vi "Import OBJ.vi"(8 "error in (no error)":errorcluster, 11 "Object":path) -> (0 "error out":errorcluster, 3 "Object":T8 {"Triangles"."Vertex 3"."UV"."v" min=0 max=1 step=0.1; "Triangles"."Vertex 3"."UV"."u" min=0 max=1 step=0.1; "Triangles"."Vertex 2"."UV"."v" min=0 max=1 step=0.1; "Triangles"."Vertex 2"."UV"."u" min=0 max=1 step=0.1; "Triangles"."Vertex 1"."UV"."v" min=0 max=1 step=0.1; "Triangles"."Vertex 1"."UV"."u" min=0 max=1 step=0.1})   [LabVIEW 2020, in "3D (FPGA).lvlib"]
uses:
  3D (FPGA).lvlib
  Vector 3D.ctl
  Object.ctl
  Transform.ctl
  Raster/UV.ctl
  Raster/Raster (FPGA).lvlib
  Vertex.ctl
  Triangle.ctl
  Raster/Rectangle Dimensions.ctl
  Raster/Texture.ctl
  Material.ctl
panel:
  out "Tris":T1[](array[typedef]) {"Vertex 3"."UV"."v" min=0 max=1 step=0.1; "Vertex 3"."UV"."u" min=0 max=1 step=0.1; "Vertex 2"."UV"."v" min=0 max=1 step=0.1; "Vertex 2"."UV"."u" min=0 max=1 step=0.1; "Vertex 1"."UV"."v" min=0 max=1 step=0.1; "Vertex 1"."UV"."u" min=0 max=1 step=0.1}
  out "text":string[](array[string])
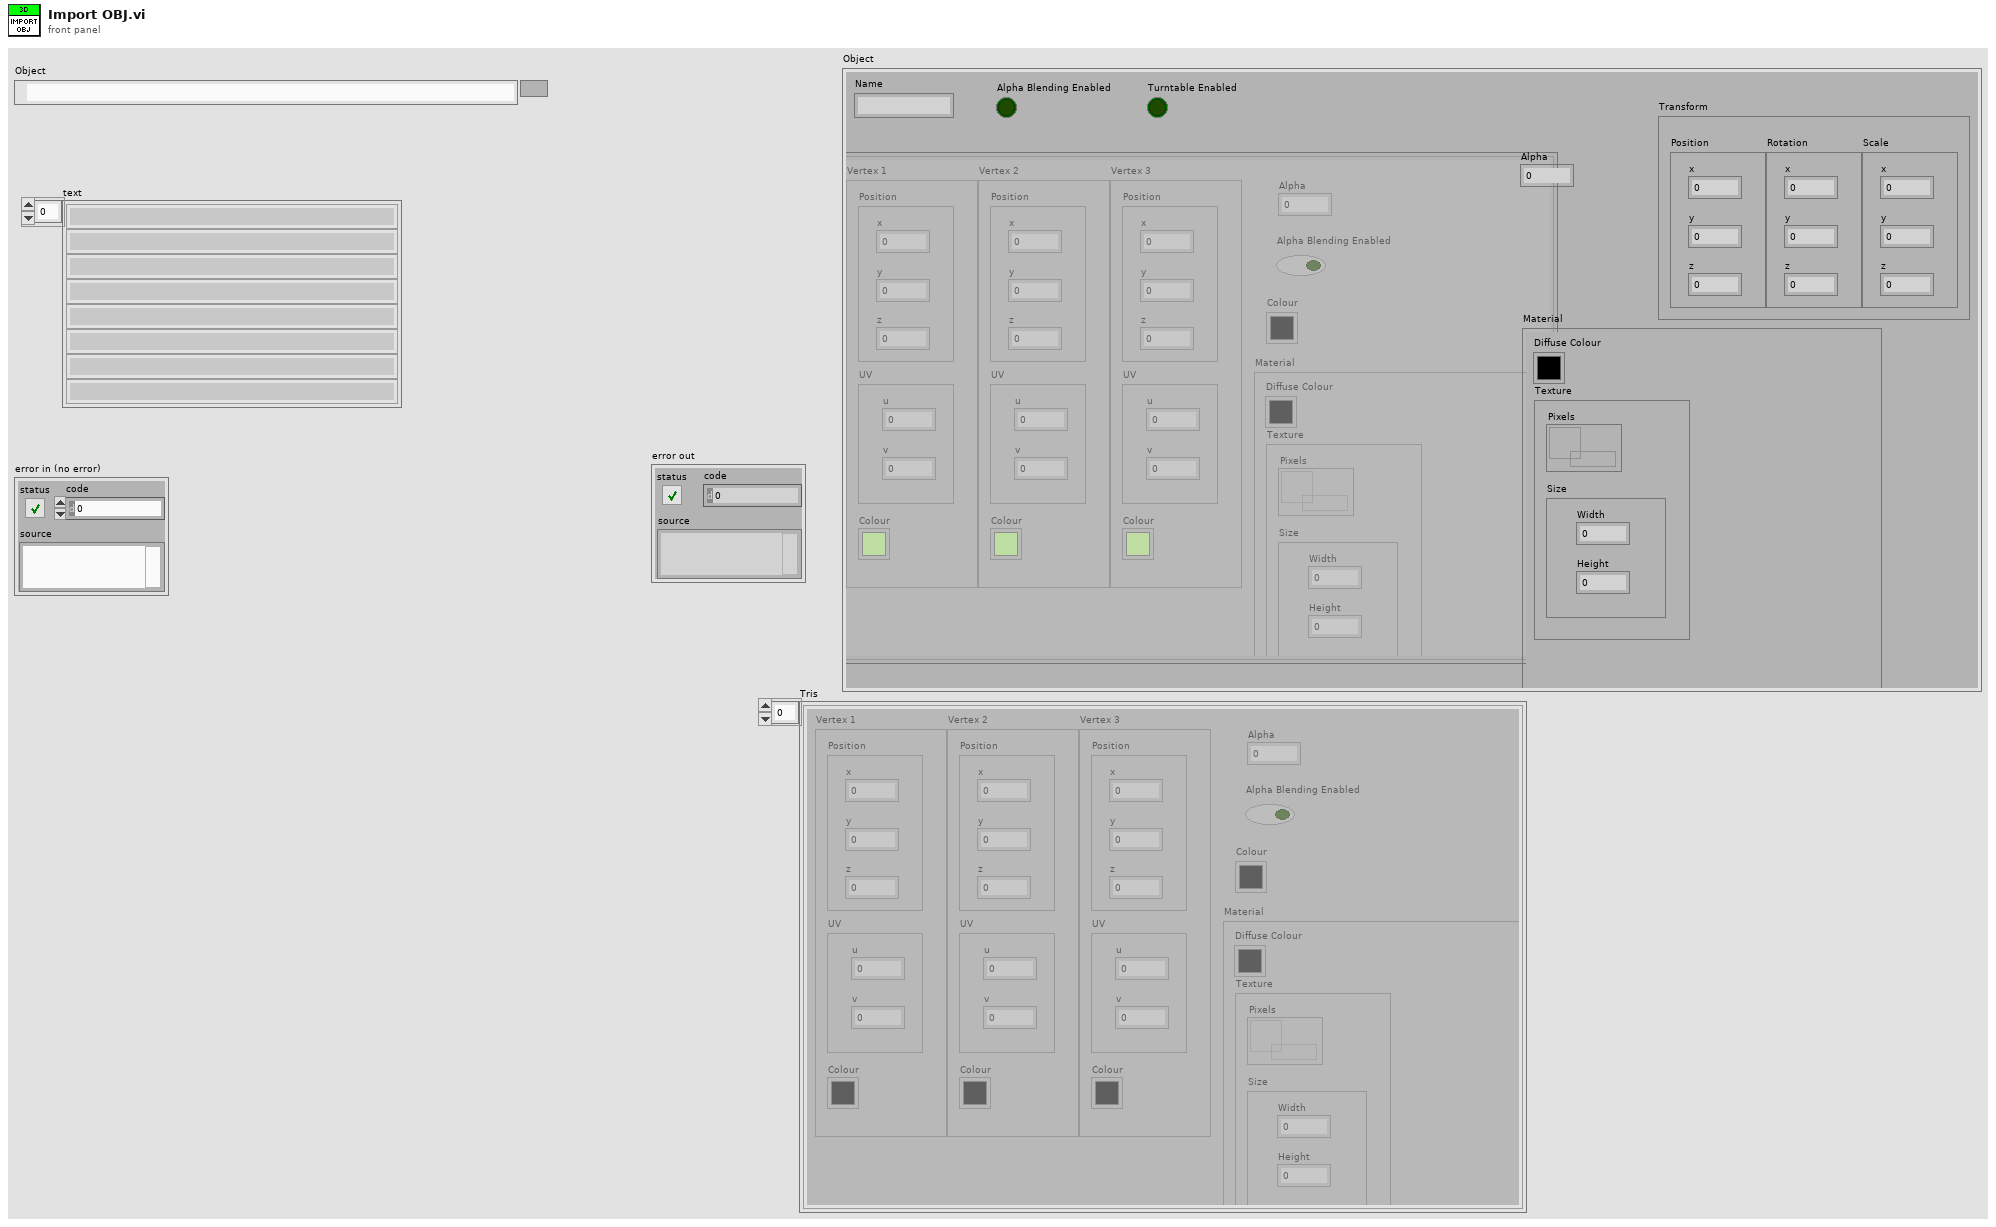
[diagram p1: front panel]
types:
  T1 = typedef "3D (FPGA).lvlib/Triangle.ctl" = cluster{"Vertex 1":T2, "Vertex 2":T2, "Vertex 3":T2, "Alpha":dbl, "Alpha Blending Enabled":bool, "Colour":u32, "Material":T5}
  T2 = typedef "3D (FPGA).lvlib/Vertex.ctl" = cluster{"Position":T3, "UV":T4, "Colour":u32}
  T3 = typedef "3D (FPGA).lvlib/Vector 3D.ctl" = cluster{"x":sgl, "y":sgl, "z":sgl}
  T4 = typedef "Raster (FPGA).lvlib/UV.ctl" = cluster{"u":sgl, "v":sgl}
  T5 = typedef "3D (FPGA).lvlib/Material.ctl" = cluster{"Diffuse Colour":u32, "Texture":T6}
  T6 = typedef "Raster (FPGA).lvlib/Texture.ctl" = cluster{"Pixels":refnum<data-value>, "Size":T7}
  T7 = typedef "Raster (FPGA).lvlib/Rectangle Dimensions.ctl" = cluster{"Width":u32, "Height":u32}
  T8 = typedef "3D (FPGA).lvlib/Object.ctl" = cluster{"Triangles":T1[], "Transform":T9, "Name":string, "Alpha Blending Enabled":bool, "Alpha":dbl, "Turntable Enabled":bool, "Material":T5}
  T9 = typedef "3D (FPGA).lvlib/Transform.ctl" = cluster{"Position":T3, "Rotation":T3, "Scale":T3}
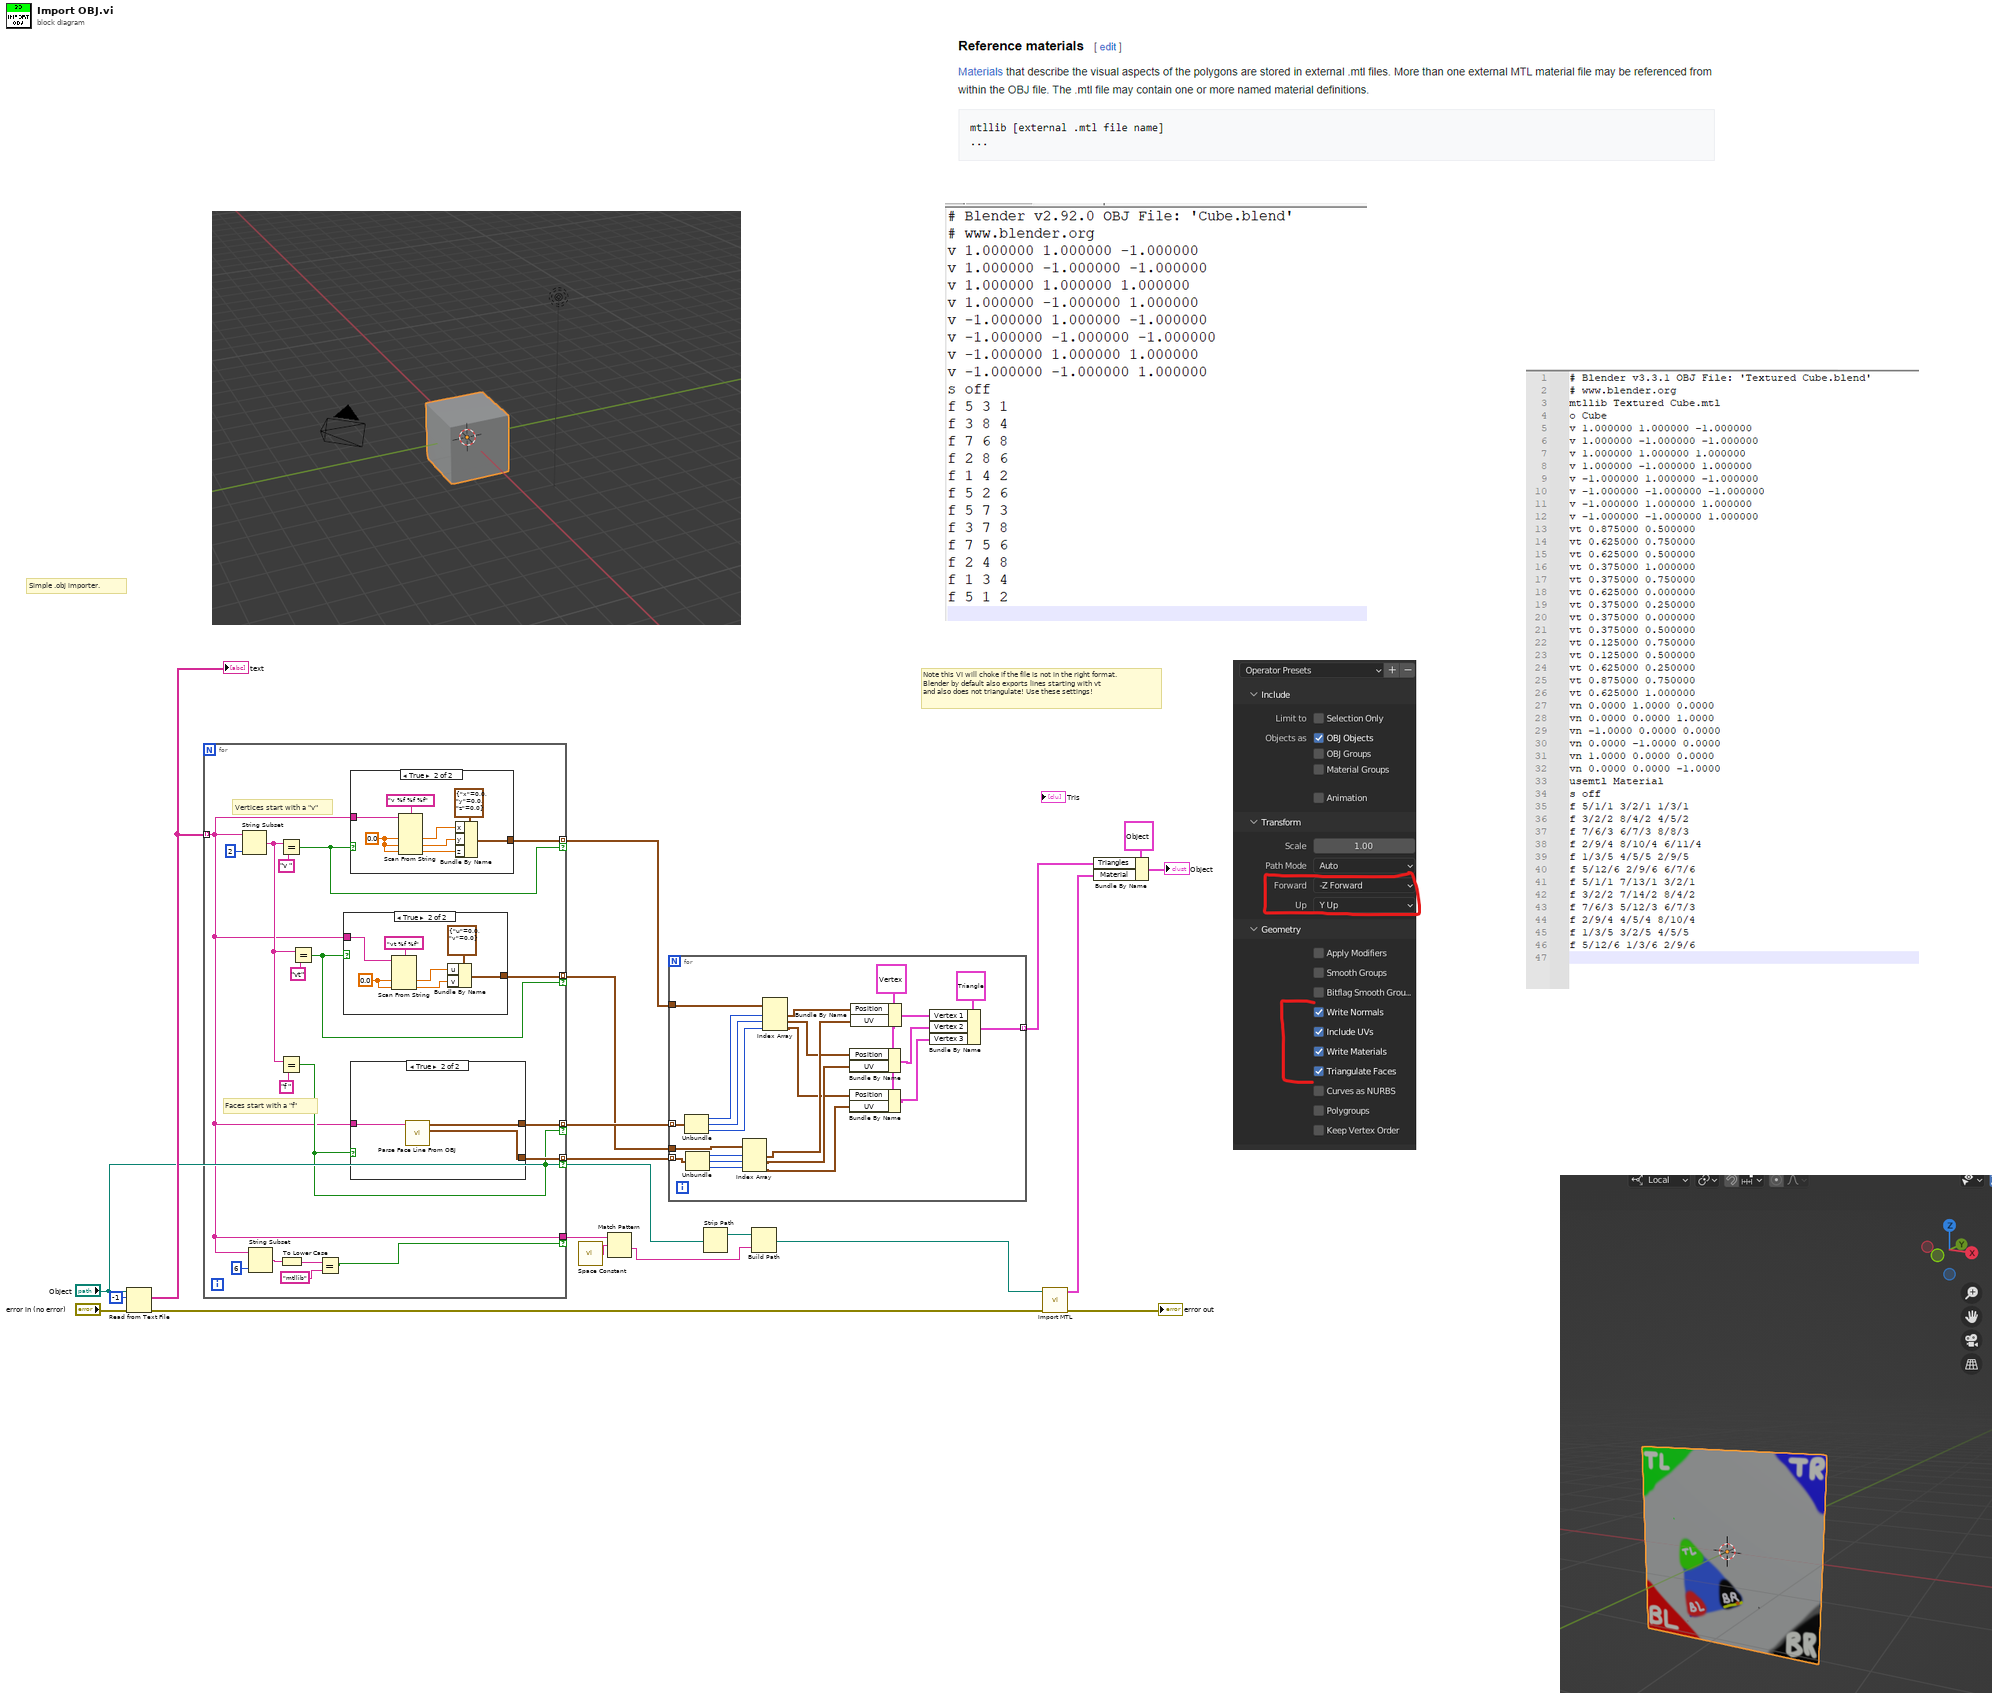
[diagram p0: block diagram]
diagram:
  # "Note this VI will choke if the file is not in the right format. Blender by default also exports lines starting with vt\nand also does not triangulate! Use these settings!"
  # "Simple .obj importer."
  n1 = Read from Text File(file (use dialog)="Object", count=-1, error in="error in (no error)") -> (text=w7:string[], error out=w10:errorcluster)  [unwired: 1 in, 2 out]
  "text" <- w7
  n2 = for {
    tunnel: w7 -> [w21] mode=indexing
    tunnel: [w34] -> w17 mode=indexing if=w33
    tunnel: [w32] -> w18 mode=indexing if=w27
    tunnel: [w29] -> w11 mode=indexing if=w26
    tunnel: [w28] -> w12 mode=indexing if=w27
    tunnel: [w21] -> w5 if=w20
    # "Faces start with a \"f\""
    # "Vertices start with a \"v\""
    n3 = String Subset(string=w21, length (rest)=2 ("length (rest)")) -> (substring=w30:string)  [unwired: 1 in]
    n4 = String Subset(string=w21, length (rest)=6 ("length (rest)")) -> (substring=w24:string)  [unwired: 1 in]
    n5 = Equal?(x=w30, y="v ") -> (x = y?=w33:bool)
    n6 = Equal?(x=w30, y="f ") -> (x = y?=w27:bool)
    n7 = To Lower Case(string=w24) -> (all lower case string=w22:string)
    n8 = Equal?(x=w30, y="vt") -> (x = y?=w26:bool)
    n9 = Equal?(x=w22, y="mtllib") -> (x = y?=w20:bool)
    n10 = case shown="True" w26 {
      tunnel: [_ w40] -> w29
      tunnel: w21 -> [_ w39]
      frame False {
      }
      frame True {
        w43 = sgl 0.0 ("default value 1")
        n11 = Scan From String(format string="vt %f %f", input string=w39, default 1=w43, default 2=w43) -> (output 1=w42:sgl, output 2=w41:sgl)  [unwired: 2 in, 3 out]
        n12 = Bundle By Name(cluster=T4 {"u"=0.0, "v"=0.0} ("Point 1"), "u"=w42, "v"=w41) -> (w40:T4)
      }
    }
    n13 = case shown="True" w33 {
      tunnel: w21 -> [_ w55]
      tunnel: [_ w48] -> w34
      frame False {
      }
      frame True {
        w53 = sgl 0.0 ("default value 1")
        n14 = Scan From String(format string="v %f %f %f", input string=w55, default 1=w53, default 2=w53, default 3=w53) -> (output 1=w51:sgl, output 2=w50:sgl, output 3=w49:sgl)  [unwired: 2 in, 3 out]
        n15 = Bundle By Name(cluster=T3 {"x"=0.0, "y"=0.0, "z"=0.0} ("Point 1"), "x"=w51, "y"=w50, "z"=w49) -> (w48:T3)
      }
    }
    n16 = case shown="True" w27 {
      tunnel: [_ w47] -> w32
      tunnel: w21 -> [_ w46]
      tunnel: [_ w45] -> w28
      frame False {
      }
      frame True {
        n17 = call "Parse Face Line From OBJ.vi"("Face string"=w46) -> ("Texture Index"=w45:cluster{"x":i32, "y":i32, "z":i32}, "Vertex Index"=w47:cluster{"x":i32, "y":i32, "z":i32})  [unwired: 8 in, 1 out]
      }
    }
  }
  n18 = call <vilib>:"Space Constant.vi"() -> ("String"=w6:string)
  n19 = Match Pattern(string=w5, regular expression=w6) -> (after substring=w2:string)  [unwired: 1 in, 3 out]
  n20 = for {
    tunnel: w18 -> [w77] mode=indexing
    tunnel: w17 -> [w75]
    tunnel: [w71] -> w14 mode=indexing
    tunnel: w12 -> [w67] mode=indexing
    tunnel: w11 -> [w68]
    w62 = T2 {"Position"={"x"=0.0, "y"=0.0, "z"=0.0}, "UV"={"u"=0.0, "v"=0.0}, "Colour"=12517256} ("Vertex 1")
    n21 = Unbundle(w77) -> ("x"=w74:i32, "y"=w73:i32, "z"=w72:i32)
    n22 = Unbundle(w67) -> ("x"=w66:i32, "y"=w65:i32, "z"=w64:i32)
    n23 = Index Array(array=w68, index #1=w66, index #2=w65, index #3=w64) -> (element #1=w63:T4, element #2=w59:T4, element #3=w58:T4)
    n24 = Index Array(array=w75, index #1=w74, index #2=w73, index #3=w72) -> (element #1=w69:T3, element #2=w57:T3, element #3=w56:T3)
    n25 = Bundle By Name(cluster=w62, "Position"=w57, "UV"=w59) -> (w61:T2)
    n26 = Bundle By Name(cluster=w62, "Position"=w56, "UV"=w58) -> (w60:T2)
    n27 = Bundle By Name(cluster=w62, "Position"=w69, "UV"=w63) -> (w70:T2)
    n28 = Bundle By Name(cluster=T1 {"Vertex 1"={"Position"={"x"=0.0, "y"=0.0, "z"=0.0}, "UV"={"u"=0.0, "v"=0.0}, "Colour"=12517256}, "Vertex 2"={"Position"={"x"=0.0, "y"=0.0, "z"=0.0}, "UV"={"u"=0.0, "v"=0.0}, "Colour"=12517256}, "Vertex 3"={"Position"={"x"=0.0, "y"=0.0, "z"=0.0}, "UV"={"u"=0.0, "v"=0.0}, "Colour"=12517256}, "Alpha"=0.0, "Alpha Blending Enabled"=FALSE, "Colour"=0, "Material"={"Diffuse Colour"=0, "Texture"={"Pixels"=refnum, "Size"={"Width"=0, "Height"=0}}}} ("Cluster"), "Vertex 1"=w70, "Vertex 2"=w61, "Vertex 3"=w60) -> (w71:T1)
  }
  n29 = Strip Path(path="Object") -> (stripped path=w3:path)  [unwired: 1 out]
  n30 = Build Path(base path=w3, name or relative path=w2) -> (appended path=w1:path)
  n31 = call "Import MTL.vi"("error in (no error)"=w10, "Material"=w1) -> ("error out"=→"error out":errorcluster, "Material"=w8:T5)  [unwired: 8 in]
  n32 = Bundle By Name(cluster=T8 {"Triangles"=[], "Transform"={"Position"={"x"=0.0, "y"=0.0, "z"=0.0}, "Rotation"={"x"=0.0, "y"=0.0, "z"=0.0}, "Scale"={"x"=0.0, "y"=0.0, "z"=0.0}}, "Name"="", "Alpha Blending Enabled"=FALSE, "Alpha"=0.0, "Turntable Enabled"=FALSE, "Material"={"Diffuse Colour"=0, "Texture"={"Pixels"=refnum, "Size"={"Width"=0, "Height"=0}}}} ("Object"), "Triangles"=w14, "Material"=w8) -> (→"Object":T8)
